vi "check angle-distance.vi"() -> ()   [LabVIEW 2019]
panel:
  out "deg":dbl[](graph)
  out "slope":dbl[](graph)
  out "distance":dbl[](graph)
  in  "Lidar data":cluster{"x":sgl, "y":sgl}[](graph)
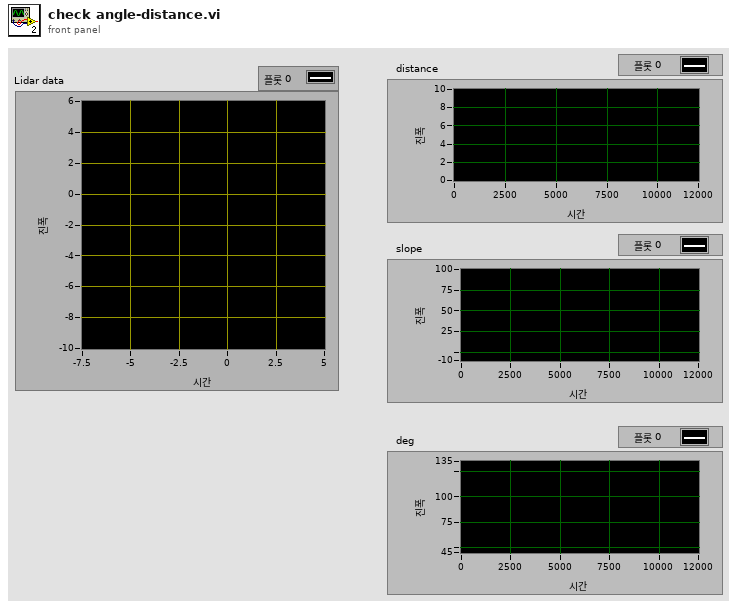
[diagram p1: front panel]
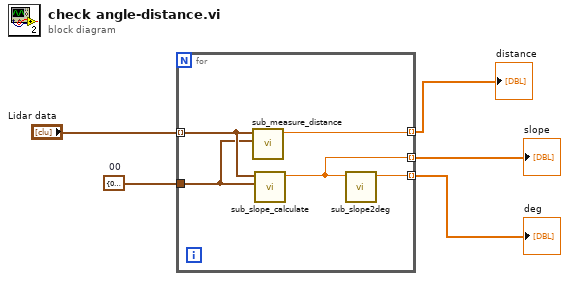
[diagram p0: block diagram]
diagram:
  w4 = cluster{"x":dbl, "y":dbl} {"x"=0.0, "y"=0.0}  # 00
  n1 = for {
    tunnel: "Lidar data" -> [w10] mode=indexing
    tunnel: w4 -> [w9]
    tunnel: [w8] -> w1 mode=indexing
    tunnel: [w7] -> w2 mode=indexing
    tunnel: [w6] -> w3 mode=indexing
    n2 = call "sub_measure_distance.vi"("pt 2"=w9, "pt 1"=w10) -> ("distance"=w6:dbl)  [unwired: 9 in]
    n3 = call "sub_slope_calculate.vi"("point n+1"=w9, "point n"=w10) -> ("slope"=w7:dbl)  [unwired: 7 in, 2 out]
    n4 = call "sub_slope2deg.vi"("slope"=w7) -> ("deg"=w8:dbl)  [unwired: 10 in]
  }
  "distance" <- w3
  "slope" <- w2
  "deg" <- w1
